vi "SPU_Waiting_for_sampling.vi"(7 "错误输入（无错误）":errorcluster, 10 "引用":refnum<k24>) -> (0 "error IO":errorcluster, 3 "引用输出":refnum<k24>)   [LabVIEW 2017]
doc: "SPU waiting for sampling"
uses:
  D:/test/PDLSTS/LV_PDL_Sample/DLL/InstrumentDLL.dll
  DLL/InstrumentDLL.dll
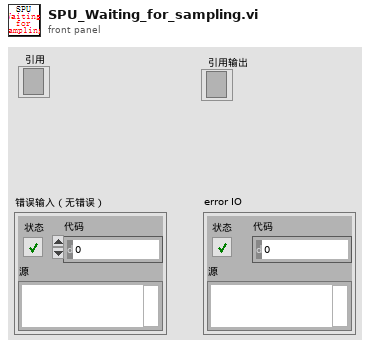
[diagram p1: front panel]
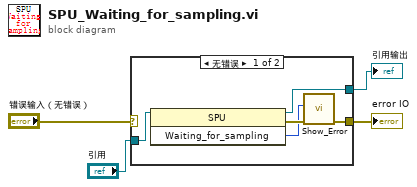
[diagram p0: block diagram]
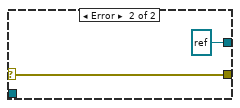
[diagram p2: hidden frame]
diagram:
  n1 = case shown="无错误" "错误输入（无错误）" {
    selector: "错误输入（无错误）" -> [_ w11]
    tunnel: [w7 w11] -> w2
    tunnel: [w6 refnum<k24> refnum ("new reference")] -> w3
    tunnel: "引用" -> [w5 _]
    frame No Error {
      n2 = invoke class="SPU" method="Waiting_for_sampling"(reference=w5) -> (reference out=w6:refnum<k24>, error out=w9:errorcluster, "Waiting_for_sampling"=w8:i32)  [unwired: 2 in]
      n3 = call "Show_Error.vi"("error in (no error)"=w9, "Error"=w8) -> ("error out"=w7:errorcluster)  [unwired: 9 in]
    }
    frame Error {
    }
  }
  "引用输出" <- w3
  "error IO" <- w2
